vi "WriteTranslateMeToDictionary.vi"() -> ()   [LabVIEW 2017]
uses:
  src/API/JKI Simple Localization.lvlib
  src/Definitions/Private/FontCluster.ctl
panel:
  in  "Fonts":T1[](array[typedef])=[{"Language"="English", "Name"="Roboto Light", "Color"=3947580}, {"Language"="Dutch", "Name"="Roboto Light", "Color"=3947580}, {"Language"="Chinese", "Name"="SimSun", "Color"=3947580}]
  out "error out":errorcluster
  in  "Dictionary Path":path
  out "Text Written":string
  in  "Additional Languages":string[](array[string])
  in  "Current VI Language":string
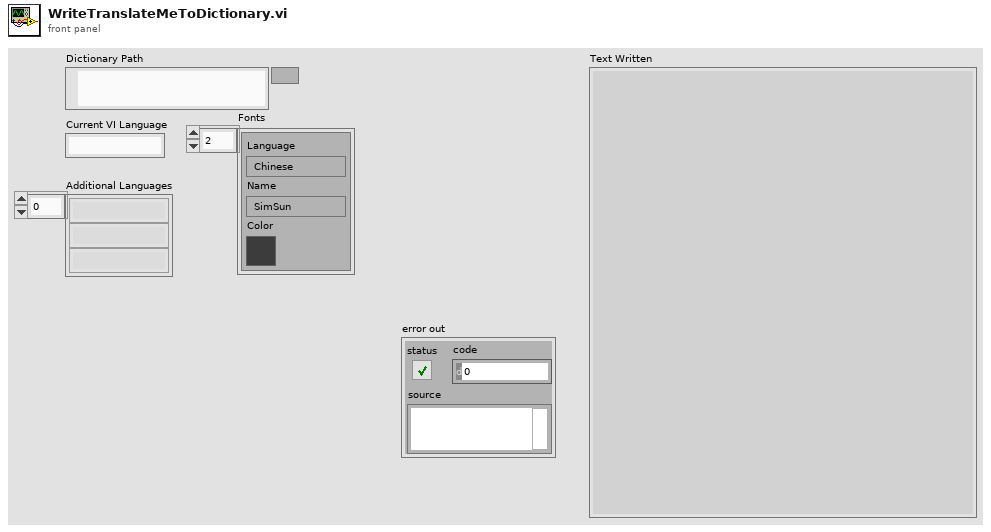
[diagram p1: front panel]
types:
  T1 = typedef "JKI Simple Localization.lvlib/FontCluster.ctl" = cluster{"Language":string, "Name":string, "Color":u32}
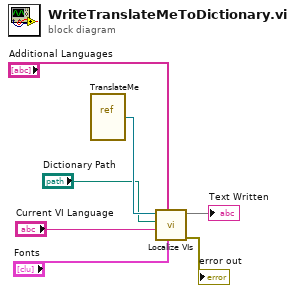
[diagram p0: block diagram]
diagram:
  n1 = vi-ref "TranslateMe.vi"() -> (w7:refnum<vi>)
  n2 = call "Localize VIs.vi"("Prompt user for new dictionary languages? (T)"="Fonts", 7:"Additional Languages", 9:"Current VI Language", "Dictionary Path"="Dictionary Path", "VIs in"=w7) -> ("error out"=→"error out":errorcluster, 3:→"Text Written")  [unwired: 5 in]
